vi "Load All Config Data.vi"(4 "error in (no error)":errorcluster, 7 "path":path=path "C:/Users/Public/SSDC/genappmainrepos/Project/ConfigdB/Config.db3") -> (0 "error out":errorcluster)   [LabVIEW 2023]
doc: "[Ver 1.00]\nDESCRIPTION\nLoad all configuration data from the ini file\n\nERROR HANDLING\nThrow, log error\n\n------------------------------------------------------------------------\n[Ver 1.00]\nSWatts SSDC 7/4/03"
uses:
  Error/ErrorCommand.ctl
  ConfigCommand.ctl
  Database/SystemdBCommands.ctl
panel:
  # "Output"
  # "Input"
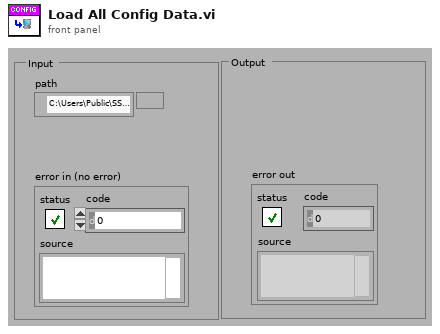
[diagram p1: front panel]
types:
  T1 = typedef "SystemdBCommands.ctl" = enum16{"No Command - Error", "Set Filepath", "Connect dB", "Disconnect dB", "Start Transaction", "Commit", "Rollback", "Describe Table", "Select All From Table", "Fetch Query", "Count Records In Table", "Get User Information", "Get System Config", "Insert New System Config", "UPDATE User Info", "Insert New User", "Get Versions", "Update Key", "Set Version to Default", "Get Default Version", "INSERT Error", "UPDATE Error", "DELETE Errors", "Get All Errors", "Get #Errors for Error"}
  T2 = typedef "ConfigCommand.ctl" = enum16{"No Command - Error", "Initialise Config SQLite", "Save Config", "Get Key", "Set Key", "Update Key", "Get Latest Config Data", "Get Config Data for Version", "Get Default Config Data"}
  T3 = typedef "ErrorCommand.ctl" = enum16{"No Command - Error", "Set to Dev Mode", "Set To Released Mode", "Set Error", "Log Error", "Throw Error", "Log & Throw Error", "Set Error Timed"}
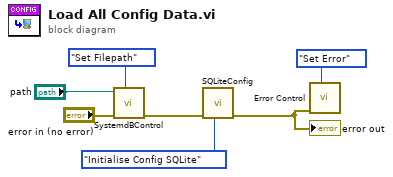
[diagram p0: block diagram]
diagram:
  n1 = call "SystemdBControl.vi"("Command"=SystemdBCommands."Set Filepath", "error in (no error)"="error in (no error)", "Data In"="path") -> ("error out"=w2:errorcluster)  [unwired: 4 in, 2 out]
  n2 = call "SQLiteConfig.vi"("ConfigCommand"=ConfigCommand."Initialise Config SQLite", "error in (no error)"=w2) -> ("error out"=w5:errorcluster)  [unwired: 3 in, 3 out]
  "error out" <- w5
  n3 = call "Error Control.vi"("Command"=ErrorCommand."Set Error", "error in (no error)"=w5) -> ()  [unwired: 6 in, 1 out]
